vi "GetLCDResultNames.vi"(7 "ProjectName":string="Prj", 10 "Analysis_LCD_Parameter":T1={"ROI"={"Global Rectangle"=[27, 55, 270, 147], "Contours"=[{"Contour Type"=0, "ROI Type"=3, "Points"=[27, 55, 270, 147]}]}, "Number of Matches Requested"=1} {"Number of Matches Requested" min=1 max=9999}, 11 "ROI_Name":string="ROI1") -> (3 "ResultNames":string[](array[string]))   [LabVIEW 2015]
uses:
  Controls/LCD/Analysis_LCD_Result.ctl
  Controls/LCD/Analysis_LCD_Parameter.ctl
panel:
  out "Array Element.Value":variant
  in  "Analysis_LCD_Result":T2={"ROI"={"Global Rectangle"=[27, 55, 270, 147], "Contours"=[{"Contour Type"=0, "ROI Type"=3, "Points"=[27, 55, 270, 147]}]}, "Output value"=0.0}
  out "error out":errorcluster
  in  "error in (no error)":errorcluster
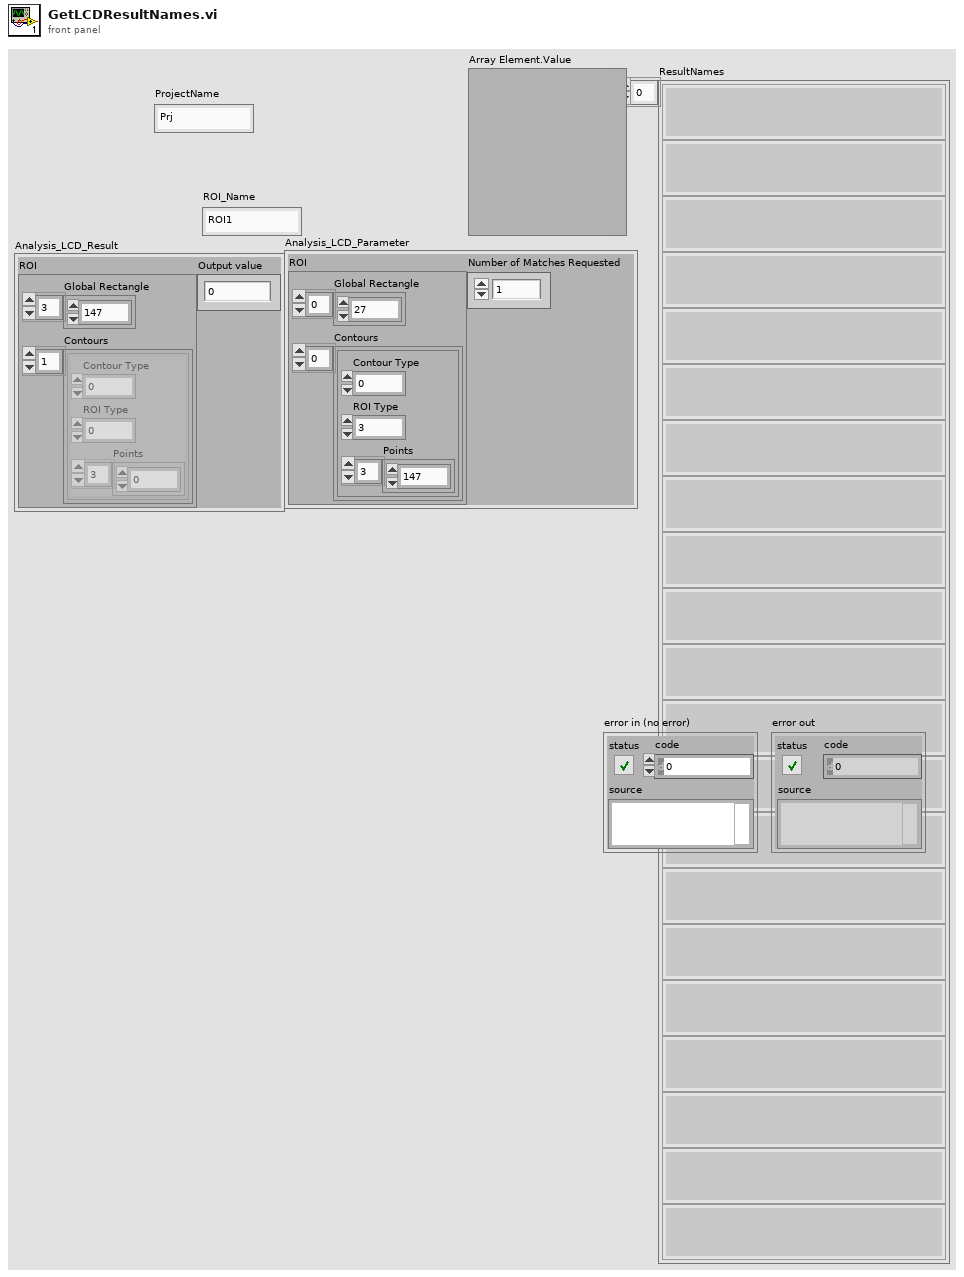
[diagram p1: front panel]
types:
  T1 = typedef "Analysis_LCD_Parameter.ctl" = cluster{"ROI":cluster{"Global Rectangle":i32[], "Contours":cluster{"Contour Type":u32, "ROI Type":u32, "Points":i32[]}[]}, "Number of Matches Requested":i32}
  T2 = typedef "Analysis_LCD_Result.ctl" = cluster{"ROI":cluster{"Global Rectangle":i32[], "Contours":cluster{"Contour Type":u32, "ROI Type":u32, "Points":i32[]}[]}, "Output value":dbl}
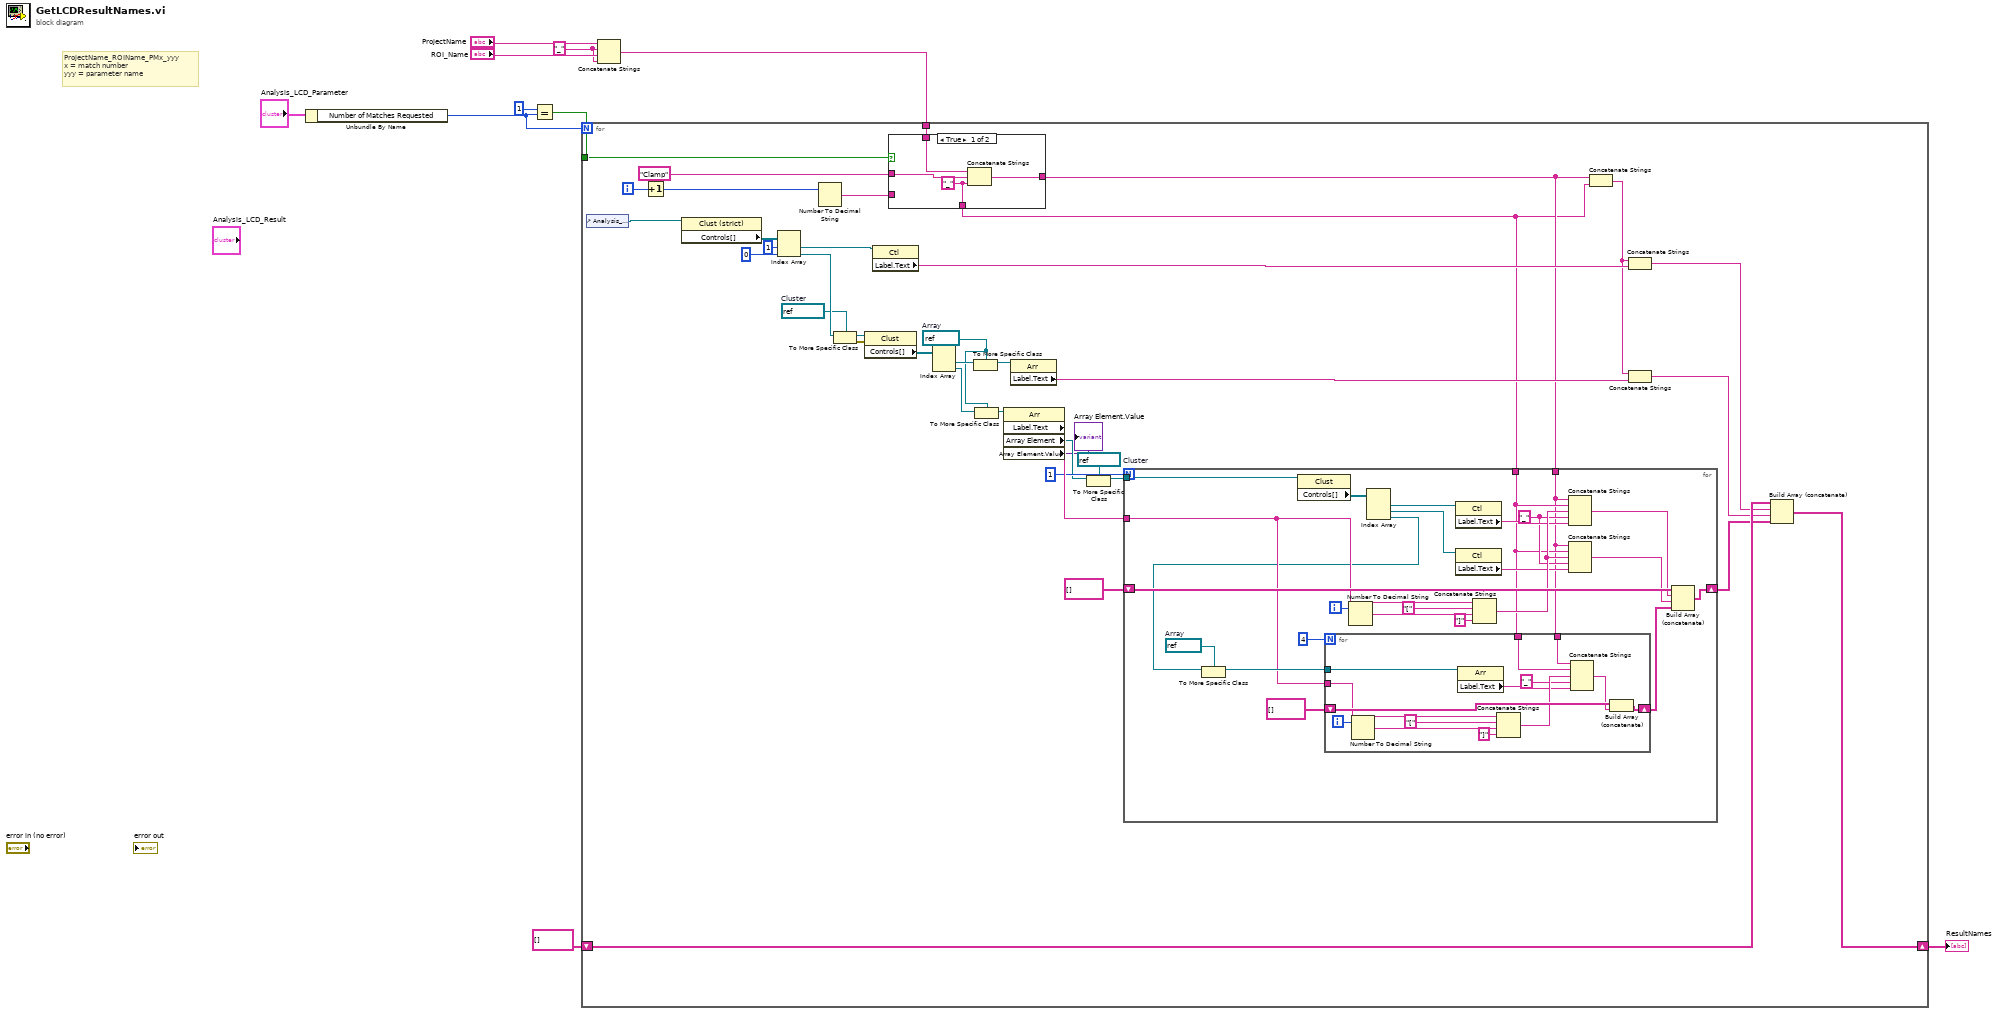
[diagram p0: block diagram]
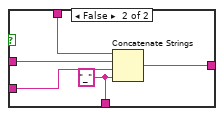
[diagram p2: hidden frame]
diagram:
  w7 = "_" ("string")
  # "ProjectName_ROIName_PMx_yyy\nx = match number\nyyy = parameter name"
  n1 = Unbundle By Name("Analysis_LCD_Parameter") -> ("Number of Matches Requested"=w1:i32)
  n2 = Equal?(x=1, y=w1) -> (x = y?=w3:bool)
  n3 = Concatenate Strings("ProjectName", w7, "ROI_Name", w7) -> (w6:string)
  n4 = for {
    N: w1 -> [_]
    tunnel: w6 -> [w46]
    shift-right: [w39] -> w4
    shift-left: string[] [] -> [w42]
    tunnel: w3 -> [w47]
    i -> [w43]
    w16 = refnum<vi> refnum  # Cluster
    w23 = refnum<vi> refnum  # Array
    w32 = refnum<vi> refnum  # Cluster
    n5 = control-ref of="Analysis_LCD_Result"() -> (w34:refnum<vi>)
    n6 = Increment(x=w43) -> (x+1=w48:i32)
    n7 = property class="Clust (strict)"(reference=w34) -> ("Controls[]"=w41:refnum<vi>[])  [unwired: 1 in, 2 out]
    n8 = Index Array(array=w41, index #1=1 ("index"), index #2=0) -> (element #1=w37:refnum<vi>, element #2=w33:refnum<vi>)
    n9 = Number To Decimal String(number=w48) -> (decimal integer string=w45:string)  [unwired: 1 in]
    n10 = To More Specific Class(target class=w32, reference=w33) -> (specific class reference=w31:refnum<vi>, error out=w30:errorcluster)  [unwired: 1 in]
    n11 = property class="Clust"(reference=w31, error in=w30) -> ("Controls[]"=w29:refnum<vi>[])  [unwired: 2 out]
    n12 = property class="Ctl"(reference=w37) -> ("Label.Text"=w36:string)  [unwired: 1 in, 2 out]
    n13 = case shown="True" w47 {
      tunnel: w46 -> [w91 w96]
      tunnel: w45 -> [_ w94]
      tunnel: [w90 w95] -> w19
      tunnel: "Clamp" ("string") -> [w89 w93]
      tunnel: [w88 w92] -> w18
      frame True {
        w88 = "_" ("string")
        n14 = Concatenate Strings(w91, w89, w88) -> (w90:string)
      }
      frame False {
        w92 = "_" ("string")
        n15 = Concatenate Strings(w96, w93, w94, w92) -> (w95:string)
      }
    }
    n16 = Index Array(array=w29) -> (element #1=w25:refnum<vi>, element #2=w24:refnum<vi>)  [unwired: 2 in]
    n17 = To More Specific Class(target class=w23, reference=w25) -> (specific class reference=w28:refnum<vi>)  [unwired: 1 in, 1 out]
    n18 = To More Specific Class(target class=w23, reference=w24) -> (specific class reference=w20:refnum<vi>)  [unwired: 1 in, 1 out]
    n19 = property class="Arr"(reference=w20) -> ("Label.Text"=w21:string, "Array Element"=w12:refnum<vi>, "Array Element.Value"=→"Array Element.Value":variant)  [unwired: 1 in, 2 out]
    n20 = property class="Arr"(reference=w28) -> ("Label.Text"=w27:string)  [unwired: 1 in, 2 out]
    n21 = To More Specific Class(target class=w16, reference=w12) -> (specific class reference=w15:refnum<vi>)  [unwired: 1 in, 1 out]
    n22 = for {
      N: 1 -> [_]
      tunnel: w21 -> [w51]
      tunnel: w15 -> [w54]
      tunnel: w19 -> [w55]
      tunnel: w18 -> [w56]
      shift-right: [w70] -> w13
      shift-left: string[] [] -> [w73]
      i -> [w69]
      w53 = refnum<vi> refnum  # Array
      w63 = "_" ("string")
      n23 = property class="Clust"(reference=w54) -> ("Controls[]"=w62:refnum<vi>[])  [unwired: 1 in, 2 out]
      n24 = Number To Decimal String(number=w69) -> (decimal integer string=w67:string)  [unwired: 1 in]
      n25 = Index Array(array=w62) -> (element #1=w61:refnum<vi>, element #2=w59:refnum<vi>, element #3=w49:refnum<vi>)  [unwired: 3 in]
      n26 = To More Specific Class(target class=w53, reference=w49) -> (specific class reference=w52:refnum<vi>)  [unwired: 1 in, 1 out]
      n27 = for {
        N: 4 -> [_]
        tunnel: w51 -> [w81]
        tunnel: w55 -> [w87]
        tunnel: w56 -> [w86]
        shift-right: [w83] -> w50
        shift-left: string[] [] -> [w85]
        tunnel: w52 -> [w74]
        i -> [w82]
        n28 = Number To Decimal String(number=w82) -> (decimal integer string=w79:string)  [unwired: 1 in]
        n29 = property class="Arr"(reference=w74) -> ("Label.Text"=w76:string)  [unwired: 1 in, 2 out]
        n30 = Concatenate Strings(w81, "[" ("string"), w79, "]" ("string")) -> (w77:string)
        n31 = Concatenate Strings(w87, w86, w77, "_" ("string"), w76) -> (w84:string)
        n32 = Build Array (concatenate)(w85, w84) -> (w83:string[])
      }
      n33 = property class="Ctl"(reference=w61) -> ("Label.Text"=w64:string)  [unwired: 1 in, 2 out]
      n34 = property class="Ctl"(reference=w59) -> ("Label.Text"=w60:string)  [unwired: 1 in, 2 out]
      n35 = Concatenate Strings(w51, "[" ("string"), w67, "]" ("string")) -> (w65:string)
      n36 = Concatenate Strings(w55, w56, w65, w63, w64) -> (w72:string)
      n37 = Concatenate Strings(w55, w56, w65, w63, w60) -> (w71:string)
      n38 = Build Array (concatenate)(w73, w72, w71, w50) -> (w70:string[])
    }
    n39 = Concatenate Strings(w19, w18) -> (w22:string)
    n40 = Concatenate Strings(w22, w36) -> (w35:string)
    n41 = Concatenate Strings(w22, w27) -> (w26:string)
    n42 = Build Array (concatenate)(w42, w35, w26, w13) -> (w39:string[])
  }
  "ResultNames" <- w4
